vi "AutoShifting.vi"(0 "LeftPWM":dbl, 1 "AutoShift":bool, 2 "ForceHigh":bool, 3 "ForceLow":bool, 5 "RightPWM":dbl, 7 "Wheel Speed":dbl, 9 "LinearPower":dbl, 11 "Throttle":dbl) -> (8 "isHighGear":bool)   [LabVIEW 2014]
uses:
  <vilib>/addons/control/pid/pid.llb/PID Control Input Filter (DBL).vi
  <vilib>/addons/control/pid/NI_PID_pid.lvlib
panel:
  in  "Voltage Threshold":dbl=9.0
  in  "Wheel Low Accel threshold":dbl=-1.0
  in  "Low Speed Threshold":dbl=5.0
  in  "WheelAccelThreshold":dbl=1.0
  in  "ThrottleAccelThreshold":dbl=0.1
  in  "Throttle Threshold":dbl=0.6
  in  "Hysterisis":i32=500
  in  "TurnThreshold":dbl=0.5
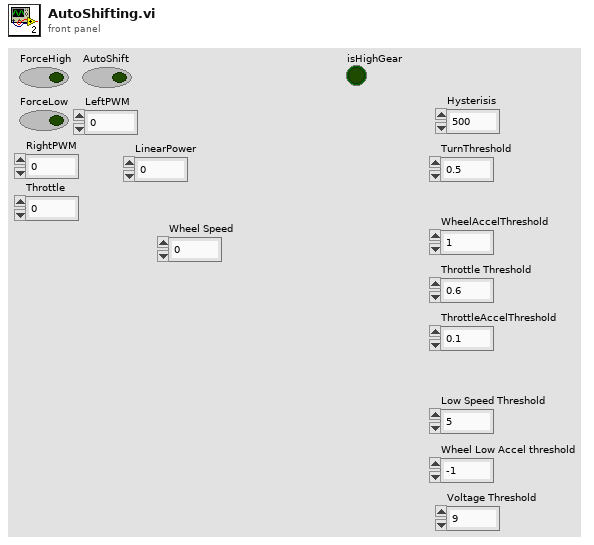
[diagram p1: front panel]
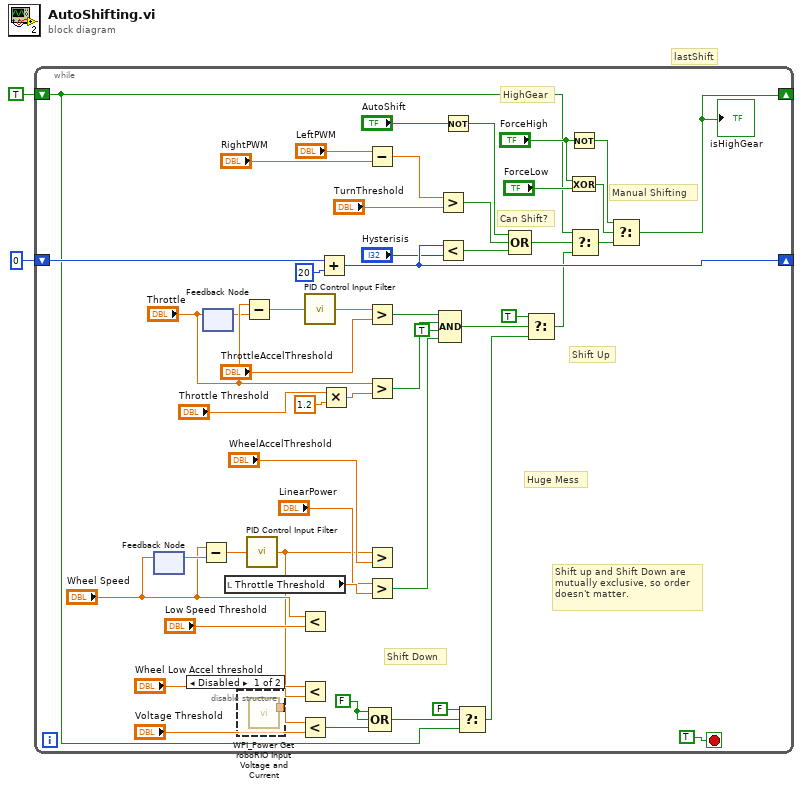
[diagram p0: block diagram]
diagram:
  # "lastShift"
  n1 = while {
    shift-right: [w37] -> _
    shift-left: 0 -> [w53]
    shift-right: [w47] -> _
    shift-left: TRUE -> [w15]
    stop <- TRUE stop-if-true
    w3 = FALSE ("t")
    # "Shift up and Shift Down are\nmutually exclusive, so order\ndoesn't matter."
    # "Shift Down"
    # "Shift Up"
    # "Can Shift?"
    # "Manual Shifting"
    # "Huge Mess"
    # "HighGear"
    n2 = feedback #1() -> (w26:dbl)  [unwired: 1 in]
    n3 = feedback-in #1("Wheel Speed") -> ()
    n4 = Subtract(x="Wheel Speed", y=w26) -> (x-y=w27:dbl)
    n5 = feedback #2() -> (w18:dbl)  [unwired: 1 in]
    n6 = feedback-in #2("Throttle") -> ()
    n7 = local read "Throttle Threshold"() -> (w29:dbl)
    n8 = disable-structure shown="Disabled" {
      disable-tunnel: [w55 _] -> w7
      frame Disabled {
        n9 = call <vilib>:"WPI_Power Get roboRIO Input Voltage and Current.vi"() -> ("roboRIO input voltage (V)"=w55:dbl)  [unwired: 13 in, 2 out]
      }
      frame Enabled {
      }
    }
    n10 = Subtract(x="Throttle", y=w18) -> (x-y=w19:dbl)
    n11 = call-poly <vilib>:"PID Control Input Filter.vi"("input"=w27) -> ("output"=w8:dbl)  [unwired: 4 in]
    n12 = Less?(x="Wheel Speed", y="Low Speed Threshold") -> ()  [unwired: 1 out]
    n13 = Less?(x="Wheel Low Accel threshold", y=w8) -> ()  [unwired: 1 out]
    n14 = Less?(x=w7, y="Voltage Threshold") -> (x < y?=w5:bool)
    n15 = call-poly <vilib>:"PID Control Input Filter.vi"("input"=w19) -> ("output"=w24:dbl)  [unwired: 4 in]
    n16 = Add(x=w53, y=20) -> (x+y=w37:i32)
    n17 = Multiply(x="Throttle Threshold", y=1.2) -> (x*y=w22:dbl)
    n18 = Subtract(x="LeftPWM", y="RightPWM") -> (x-y=w40:dbl)
    n19 = Greater?(x=w24, y="ThrottleAccelThreshold") -> (0:w30:bool)
    n20 = Greater?(x="Throttle", y=w22) -> (0:w31:bool)
    n21 = Greater?(x=w8, y="WheelAccelThreshold") -> ()  [unwired: 1 out]
    n22 = Greater?(x="LinearPower", y=w29) -> (0:w32:bool)
    n23 = Compound Arithmetic op=OR(w3, w3, w5) -> (w12:bool)
    n24 = Greater?(x=w40, y="TurnThreshold") -> (0:w39:bool)
    n25 = Less?(x=w37, y="Hysterisis") -> (x < y?=w35:bool)
    n26 = Compound Arithmetic op=AND(w30, w31, TRUE ("value"), w32) -> (w33:bool)
    n27 = Not(x="AutoShift") -> (.not. x?=w45:bool)
    n28 = Select(t=FALSE, s=w12, f=w15) -> (s? t:f=w16:bool)
    n29 = Compound Arithmetic op=OR(w45, w39, w35) -> (w44:bool)
    n30 = Select(t=TRUE, s=w33, f=w16) -> (s? t:f=w17:bool)
    n31 = Not(x="ForceHigh") -> (.not. x?=w48:bool)
    n32 = Exclusive Or(1:"ForceLow", 2:"ForceHigh") -> (0:w50:bool)
    n33 = Select(t=w15, s=w44, f=w17) -> (s? t:f=w43:bool)
    n34 = Select(t=w48, s=w50, f=w43) -> (s? t:f=w47:bool)
    "isHighGear" <- w47
  }
